vi "CC Obervation Generate Dither Step.vi"(8 "error in (no error)":errorcluster, 11 "Dither Options":T1) -> (0 "error out":errorcluster, 2 "Name":string, 3 "Step":T3={"Action"=enum."Acquire Images", "Data"=variant})   [LabVIEW 2021]
uses:
  typedefs/CC Script Step.ctl
  typedefs/CC enum Script Action.ctl
  typedefs/CC cluster Observation Dither Options.ctl
  typedefs/CC enum Dither Selection.ctl
  typedefs/CC Dithering.ctl
  typedefs/CC cluster Offset Dithering.ctl
  typedefs/CC Dithering Offsets.ctl
  typedefs/CC cluster Random Dithering.ctl
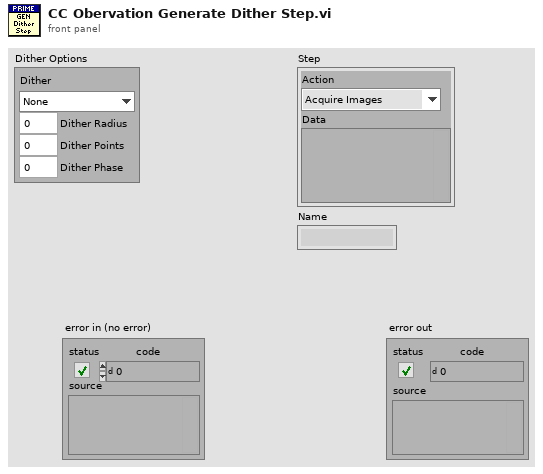
[diagram p1: front panel]
types:
  T1 = typedef "CC cluster Observation Dither Options.ctl" = cluster{"Dither":T2, "Dither Radius":dbl, "Dither Points":i32, "Dither Phase":dbl}
  T2 = typedef "CC enum Dither Selection.ctl" = enum16{"None", "Circle", "Random"}
  T3 = typedef "CC Script Step.ctl" = cluster{"Action":T4, "Data":variant}
  T4 = typedef "CC enum Script Action.ctl" = enum16{"Noop", "Define Object", "Define Exposure", "Define Dithering", "Acquire Images", "Set Filter Wheel", "Telescope Home", "Telescope Move", "Telescope RA DEC", "Focus Move Relative", "Focus Move Absolute", "Focus Set Home", "Macro", "Pause", "Ask User", "Define Random Dither"}
  T5 = typedef "CC Dithering.ctl" = cluster{"Name":string, "Dithering Offsets":T6}
  T6 = typedef "CC cluster Offset Dithering.ctl" = cluster{"Offsets":T7[]}
  T7 = typedef "CC Dithering Offsets.ctl" = cluster{"DEC":dbl, "RA":dbl}
  T8 = typedef "CC cluster Random Dithering.ctl" = cluster{"Count":i32, "Radius":dbl, "Name":string}
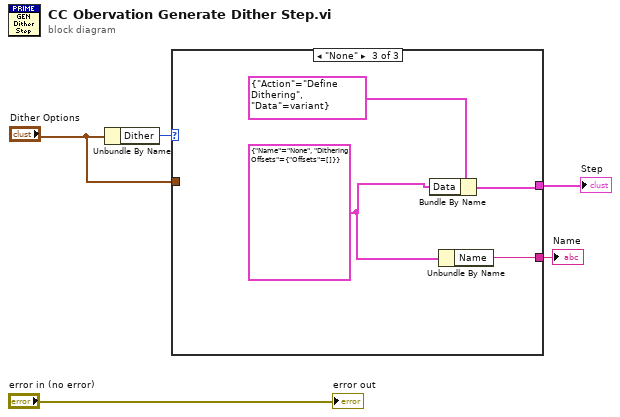
[diagram p0: block diagram]
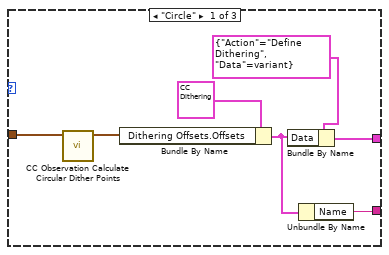
[diagram p2: hidden frame]
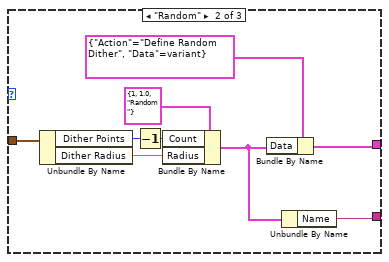
[diagram p3: hidden frame]
diagram:
  n1 = Unbundle By Name("Dither Options") -> ("Dither"=w4:T2)
  n2 = case shown="\"None\"" w4 {
    tunnel: "Dither Options" -> [w12 w20 _]
    tunnel: [w8 w16 w24] -> w2
    tunnel: [w6 w14 w23] -> w1
    frame "Circle" {
      n3 = call "CC Observation Calculate Circular Dither Points.vi"("Dither Options"=w12) -> ("Points"=w10:T7[])  [unwired: 9 in, 1 out]
      n4 = Bundle By Name(cluster=T5 {"Name"="Circle", "Dithering Offsets"={"Offsets"=[{"DEC"=-1.0, "RA"=-1.0}, {"DEC"=-1.0, "RA"=1.0}, {"DEC"=1.0, "RA"=1.0}, {"DEC"=1.0, "RA"=-1.0}]}} ("Dithering Offsets"), "Dithering Offsets.Offsets"=w10) -> (w7:T5)
      n5 = Bundle By Name(cluster=T3 {"Action"=enum."Define Dithering", "Data"=variant}, "Data"=w7) -> (w8:T3)
      n6 = Unbundle By Name(w7) -> ("Name"=w6:string)
    }
    frame "Random" {
      n7 = Unbundle By Name(w20) -> ("Dither Points"=w18:i32, "Dither Radius"=w17:dbl)
      n8 = Decrement(x=w18) -> (x-1=w13:i32)
      n9 = Bundle By Name(cluster=T8 {"Count"=1, "Radius"=1.0, "Name"="Random"} ("Random Dither"), "Count"=w13, "Radius"=w17) -> (w15:T8)
      n10 = Bundle By Name(cluster=T3 {"Action"=enum."Define Random Dither", "Data"=variant}, "Data"=w15) -> (w16:T3)
      n11 = Unbundle By Name(w15) -> ("Name"=w14:string)
    }
    frame "None" {
      w22 = T5 {"Name"="None", "Dithering Offsets"={"Offsets"=[]}} ("Dithering Offsets")
      n12 = Bundle By Name(cluster=T3 {"Action"=enum."Define Dithering", "Data"=variant}, "Data"=w22) -> (w24:T3)
      n13 = Unbundle By Name(w22) -> ("Name"=w23:string)
    }
  }
  "Step" <- w2
  "Name" <- w1
  "error out" <- "error in (no error)"
